vi "Load Bitfile Settings.vi"(8 "error in (no error)":errorcluster, 11 "bitfile path":path) -> (0 "error out":errorcluster, 1 "Bitfile Info":T1, 2 "Valid?":bool, 3 "SLSC version string":string)   [LabVIEW 2014, in "SLSC configuration System Explorer.lvlib"]
uses:
  SLSC configuration System Explorer.lvlib
  Type Defs/SLSC Bitfile Info.ctl
  Shared/Constants.vi
  Shared/SLSC configuration Shared.lvlib
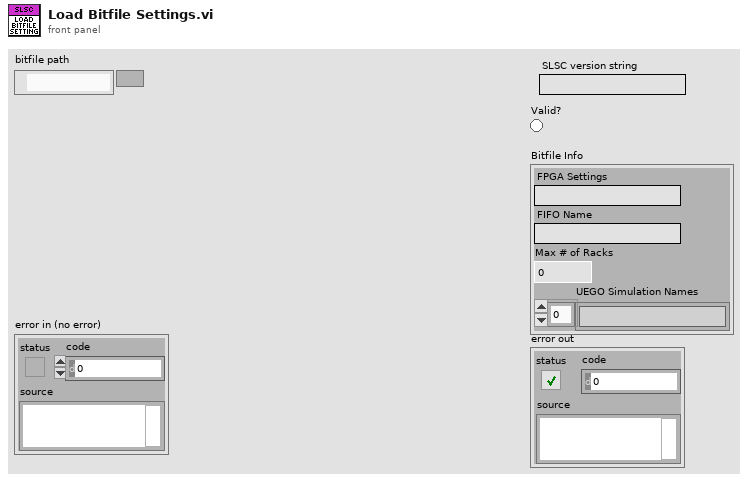
[diagram p1: front panel]
types:
  T1 = typedef "SLSC configuration System Explorer.lvlib/SLSC Bitfile Info.ctl" = cluster{"FPGA Settings":string, "FIFO Name":string, "Max # of Racks":u8, "UEGO Simulation Names":string[]}
  T2 = typedef "SLSC configuration System Explorer.lvlib/SLSC Custom Device Version.ctl" = enum8{"1.0"}
  T3 = typedef "niFpgaBitfileStructure_VI.ctl" = cluster{"Name":string, "RegisterMap":T4[], "Icon":T9}
  T4 = typedef "nirviControlStructure.ctl" = cluster{"Name":string, "Hidden":bool, "Indicator":bool, "Flattened Type":string, "Grouping":cluster{"Grouped":bool, "Member Names":string[], "Member IDs":u32[]}, "Address":u32, "Size":u32, "Class":u32, "Internal":bool, "Typedef":T5, "ID":u32, "Bidirectional":bool, "Synchronous":bool, "Mechanical Action":T6, "Sub Controls":T7[], "Access May Timeout":bool, "Register Node":bool}
  T5 = typedef "nirviTypdefDescription.ctl" = cluster{"Typedef":bool, "Path":path}
  T6 = typedef "nirviMechanicalAction.ctl" = enum8{"Switch When Pressed", "Switch When Released", "Switch Until Released", "Latch When Pressed", "Latch When Released", "Latch Until Released"}
  T7 = typedef "nirviSubControlStructure.ctl" = cluster{"Name":string, "flattened Type":string, "Cluster Information":T8, "Typedef":T5}
  T8 = typedef "nirviClusterElementControl.ctl" = cluster{"Name Hierarchy":string[], "Item Order":u32[]}
  T9 = typedef "imagedata.ctl" = cluster{"image type":i32, "image depth":i32, "image":u8[], "mask":u8[], "colors":u32[], "Rectangle":cluster{"left":i16, "top":i16, "right":i16, "bottom":i16}}
  T10 = typedef "SLSC configuration System Explorer.lvlib/Register Types.ctl" = enum16{"SLSC Settings", "# of Racks", "SPI FIFO Name", "UEGO Calibration"}
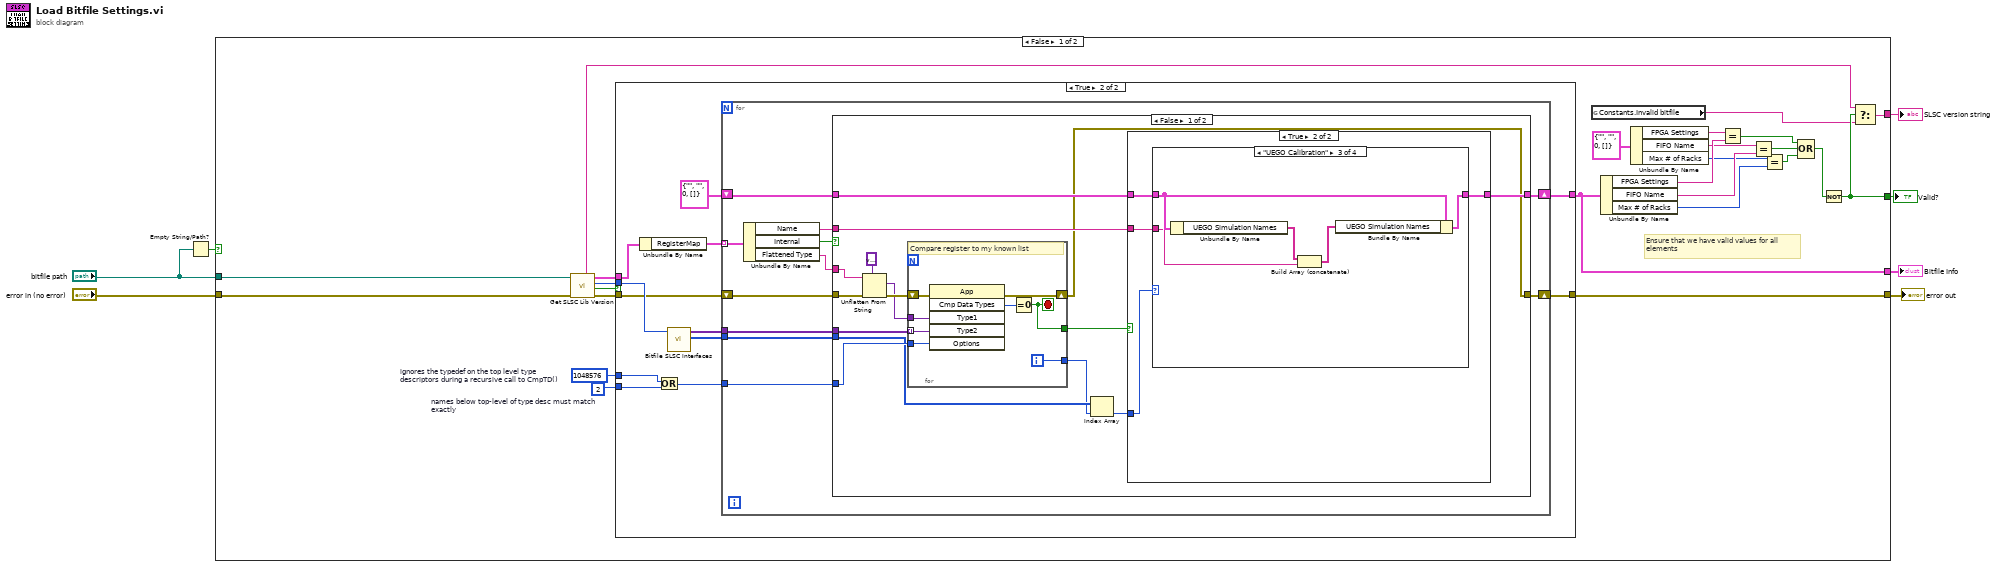
[diagram p0: block diagram]
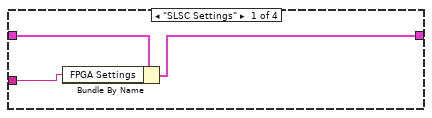
[diagram p4: hidden frame]
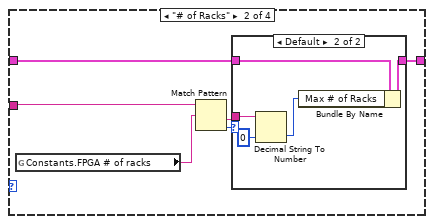
[diagram p5: hidden frame]
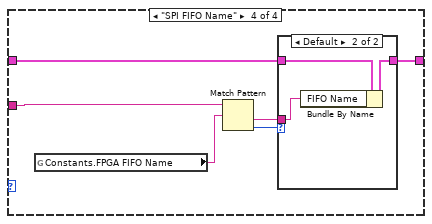
[diagram p7: hidden frame]
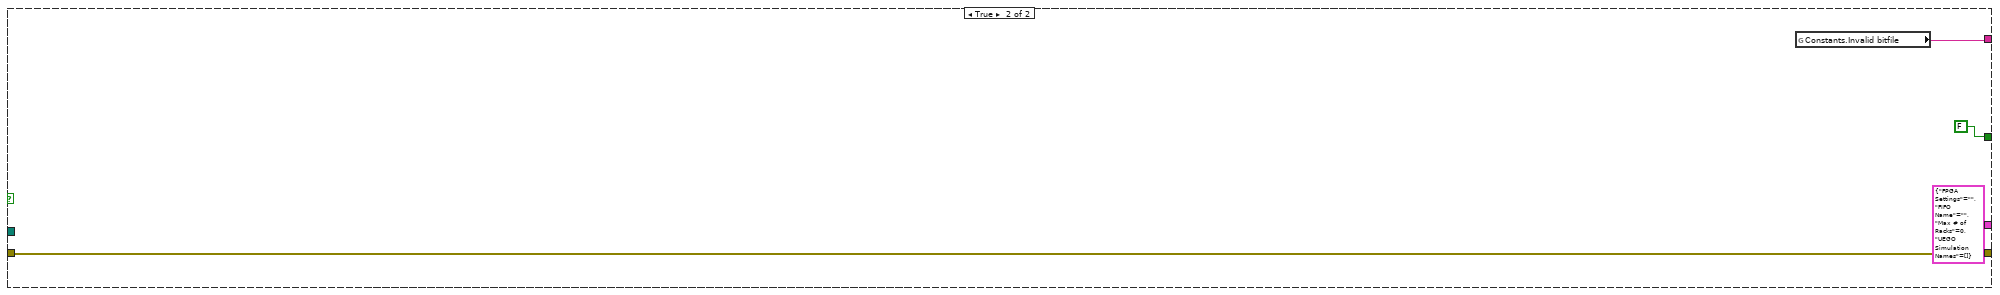
[diagram p10: hidden frame]
diagram:
  n1 = Empty String/Path?(string/path="bitfile path") -> (empty?=w1:bool)
  n2 = case shown="False" w1 {
    tunnel: [w18 T1 {"FPGA Settings"="", "FIFO Name"="", "Max # of Racks"=0, "UEGO Simulation Names"=[]} ("Cluster")] -> w7
    tunnel: "error in (no error)" -> [w26 w120]
    tunnel: [w25 w120] -> w5
    tunnel: [w24 FALSE] -> w4
    tunnel: [w21 w118] -> w3
    tunnel: "bitfile path" -> [w20 _]
    frame False {
      w27 = 2  # names below top-level of type desc must match exactly
      w28 = 1048576  # ignores the typedef on the top level type descriptors during a recursive call to CmpTD()
      # "Ensure that we have valid values for all\nelements"
      n3 = call "Get SLSC Lib Version.vi"("error in (no error)"=w26, "bitfile path"=w20) -> ("error out"=w29:errorcluster, "valid bitfile"=w32:bool, "SLSC version enum"=w31:T2, "vi info"=w30:T3, "SLSC version string"=w22:string)  [unwired: 5 in]
      n4 = case shown="True" w32 {
        tunnel: w31 -> [_ w45]
        tunnel: w30 -> [_ w44]
        tunnel: w29 -> [w33 w40]
        tunnel: w28 -> [_ w39]
        tunnel: w27 -> [_ w38]
        tunnel: [_ w35] -> w18
        tunnel: [w33 w34] -> w25
        frame False {
        }
        frame True {
          n5 = Unbundle By Name(w44) -> ("RegisterMap"=w43:T4[])
          n6 = Or(x=w39, y=w38) -> (x .or. y?=w37:i32)
          n7 = call "Bitfile SLSC Interfaces.vi"("SLSC CD Version"=w45) -> ("IP Types"=w41:T10[], "IP Interface"=w42:variant[])  [unwired: 9 in]
          n8 = for {
            tunnel: w43 -> [w56] mode=indexing
            tunnel: w42 -> [w52]
            tunnel: w41 -> [w51]
            tunnel: w37 -> [w50]
            shift-right: [w47] -> w35
            shift-left: T1 {"FPGA Settings"="", "FIFO Name"="", "Max # of Racks"=0, "UEGO Simulation Names"=[]} ("Cluster") -> [w49]
            shift-right: [w46] -> w34
            shift-left: w40 -> [w53]
            n9 = Unbundle By Name(w56) -> ("Name"=w48:string, "Internal"=w55:bool, "Flattened Type"=w54:string)
            n10 = case shown="False" w55 {
              tunnel: w54 -> [w68 _]
              tunnel: w53 -> [w67 w115]
              tunnel: w52 -> [w66 _]
              tunnel: w51 -> [w64 _]
              tunnel: w50 -> [w65 _]
              tunnel: w49 -> [w60 w116]
              tunnel: w48 -> [w59 _]
              tunnel: [w58 w116] -> w47
              tunnel: [w57 w115] -> w46
              frame False {
                n11 = Unflatten From String(type=variant ("Variant"), binary string=w68, error in (no error)=w67) -> (value=w69:variant, error out=w71:errorcluster)  [unwired: 3 out]
                n12 = for {
                  shift-right: [w113] -> w57
                  shift-left: w71 -> [w114]
                  tunnel: w69 -> [w111]
                  tunnel: w66 -> [w110] mode=indexing
                  tunnel: [w109] -> w62
                  tunnel: [w108] -> w63
                  tunnel: w65 -> [w107]
                  i -> [w108]
                  stop <- w109 stop-if-true
                  # "Compare register to my known list"
                  n13 = invoke class="App" method="Cmp Data Types"(error in=w114, "Type1"=w111, "Type2"=w110, "Options"=w107) -> (error out=w113:errorcluster, "Compare Data Types"=w112:i32)  [unwired: 2 in, 4 out]
                  n14 = Equal To 0?(x=w112) -> (x = 0?=w109:bool)
                }
                n15 = Index Array(array=w64, index=w63) -> (element=w61:T10)
                n16 = case shown="True" w62 {
                  tunnel: w61 -> [_ w76]
                  tunnel: w60 -> [w72 w75]
                  tunnel: w59 -> [_ w74]
                  tunnel: [w72 w73] -> w58
                  frame False {
                  }
                  frame True {
                    n17 = case shown="\"UEGO Calibration\"" w76 {
                      tunnel: w75 -> [w79 w82 w96 w102]
                      tunnel: w74 -> [w78 w81 w93 w100]
                      tunnel: [w77 w83 w95 w101] -> w73
                      frame "SLSC Settings" {
                        n18 = Bundle By Name(cluster=w79, "FPGA Settings"=w78) -> (w77:T1)
                      }
                      frame "# of Racks" {
                        n19 = global read "Constants.vi" "Constants.FPGA # of racks"() -> (w85:string)
                        n20 = Match Pattern(string=w81, regular expression=w85) -> (after substring=w80:string, offset past match=w84:i32)  [unwired: 1 in, 2 out]
                        n21 = case shown="Default" w84 {
                          tunnel: w82 -> [w86 w91]
                          tunnel: [w86 w90] -> w83
                          tunnel: w80 -> [_ w89]
                          frame -1 {
                          }
                          frame Default {
                            n22 = Decimal String To Number(string=w89, default (0L)=u8 0 ("default (0 I32)")) -> (number=w88:u8)  [unwired: 1 in, 1 out]
                            n23 = Bundle By Name(cluster=w91, "Max # of Racks"=w88) -> (w90:T1)
                          }
                        }
                      }
                      frame "UEGO Calibration" {
                        n24 = Unbundle By Name(w96) -> ("UEGO Simulation Names"=w94:string[])
                        n25 = Build Array (concatenate)(w94, w93) -> (w92:string[])
                        n26 = Bundle By Name(cluster=w96, "UEGO Simulation Names"=w92) -> (w95:T1)
                      }
                      frame "SPI FIFO Name" {
                        n27 = global read "Constants.vi" "Constants.FPGA FIFO Name"() -> (w98:string)
                        n28 = Match Pattern(string=w100, regular expression=w98) -> (after substring=w99:string, offset past match=w97:i32)  [unwired: 1 in, 2 out]
                        n29 = case shown="Default" w97 {
                          tunnel: w102 -> [w103 w106]
                          tunnel: [w103 w105] -> w101
                          tunnel: w99 -> [_ w104]
                          frame -1 {
                          }
                          frame Default {
                            n30 = Bundle By Name(cluster=w106, "FIFO Name"=w104) -> (w105:T1)
                          }
                        }
                      }
                    }
                  }
                }
              }
              frame True {
              }
            }
          }
        }
      }
      n31 = global read "Constants.vi" "Constants.Invalid bitfile"() -> (w23:string)
      n32 = Unbundle By Name(w18) -> ("FPGA Settings"=w16:string, "FIFO Name"=w14:string, "Max # of Racks"=w12:u8)
      n33 = Unbundle By Name(T1 {"FPGA Settings"="", "FIFO Name"="", "Max # of Racks"=0, "UEGO Simulation Names"=[]} ("Cluster")) -> ("FPGA Settings"=w17:string, "FIFO Name"=w15:string, "Max # of Racks"=w13:u8)
      n34 = Equal?(x=w17, y=w16) -> (x = y?=w11:bool)
      n35 = Equal?(x=w15, y=w14) -> (x = y?=w10:bool)
      n36 = Equal?(x=w13, y=w12) -> (x = y?=w9:bool)
      n37 = Compound Arithmetic op=OR(w11, w10, w9) -> (w8:bool)
      n38 = Not(x=w8) -> (.not. x?=w24:bool)
      n39 = Select(t=w22, s=w24, f=w23) -> (s? t:f=w21:string)
    }
    frame True {
      n40 = global read "Constants.vi" "Constants.Invalid bitfile"() -> (w118:string)
    }
  }
  "SLSC version string" <- w3
  "Bitfile Info" <- w7
  "Valid?" <- w4
  "error out" <- w5
